vi "Execute Command.vi"(7 "Execution Mode (Default: Serialized)":T1, 8 "error in (no error)":errorcluster, 10 "Command":string, 11 "Camera in":refnum<class "Camera.lvclass">) -> (0 "error out":errorcluster, 3 "Camera":refnum<class "Camera.lvclass">)   [LabVIEW 2020, in "Camera.lvclass"]
uses:
  Camera.lvclass
  Camera.lvclass/Camera.ctl
  bin/gindustrialcam_32-1.dll
  Execution Mode.ctl
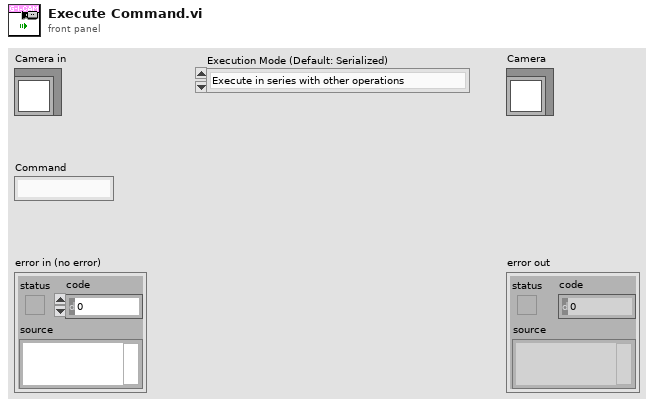
[diagram p1: front panel]
types:
  T1 = typedef "Camera.lvclass/Execution Mode.ctl" = enum16{"Execute in series with other operations", "Execute in parallel with other operations"}
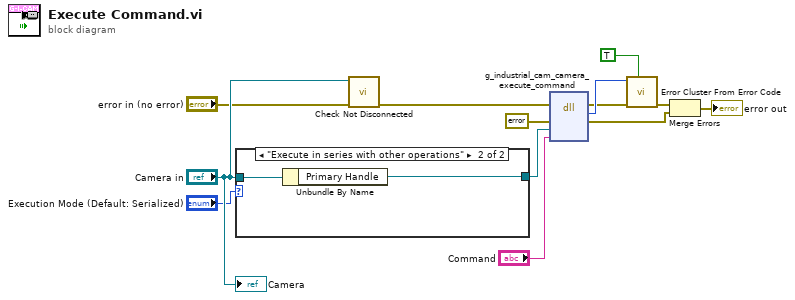
[diagram p0: block diagram]
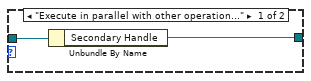
[diagram p2: hidden frame]
diagram:
  n1 = case shown="\"Execute in series with other operations\"" "Execution Mode (Default: Serialized)" {
    tunnel: "Camera in" -> [w15 w17]
    tunnel: [w14 w16] -> w9
    frame "Execute in parallel with other operations" {
      n2 = Unbundle By Name(w15) -> ("Secondary Handle"=w14:refnum<data-value>)
    }
    frame "Execute in series with other operations" {
      n3 = Unbundle By Name(w17) -> ("Primary Handle"=w16:refnum<data-value>)
    }
  }
  n4 = call "Check Not Disconnected.vi"("error in (no error)"="error in (no error)", "Camera in"="Camera in") -> ("error out"=w10:errorcluster)  [unwired: 9 in]
  n5 = dll-call lib="C:/serenial/lib/g-industrial-camera/LabVIEW/g_industrial_cam/bin/gindustrialcam_*-1.*" fn="g_industrial_cam_camera_execute_command"(error in=w10, "err"=errorcluster {"status"=FALSE, "code"=0, "source"=""} ("error constant"), "edvr"=w9, "command"="Command") -> (error out=w3:errorcluster, "Mg_Error"=w4:i32, "err"=w6:errorcluster)  [unwired: 4 in, 1 out]
  n6 = call <vilib>:"Error Cluster From Error Code.vi"("show call chain? (False)"=TRUE, "error in (no error)"=w3, "error code (0)"=w4) -> ("error out"=w5:errorcluster)  [unwired: 6 in]
  n7 = Merge Errors(w5, w6) -> (→"error out":errorcluster)
  "Camera" <- "Camera in"
